vi "obj.GetClassName.vi"(8 "error in (no error)":errorcluster, 11 "LabVIEW Object":refnum<class>) -> (0 "error out":errorcluster, 1 "name (fully qualified)":string, 2 "name (no extension)":string, 5 "is lvclass?":bool)   [LabVIEW 2020]
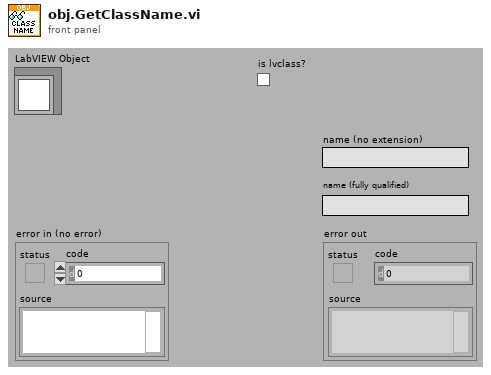
[diagram p1: front panel]
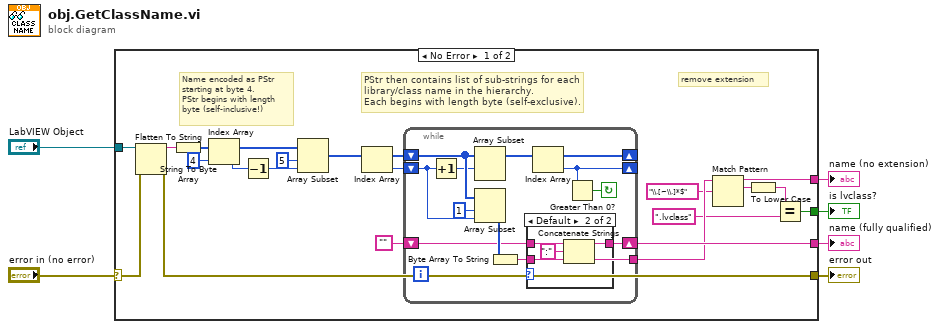
[diagram p0: block diagram]
diagram:
  n1 = case shown="No Error" "error in (no error)" {
    selector: "error in (no error)" -> [w15 w44]
    tunnel: "LabVIEW Object" -> [w26 _]
    tunnel: [w14 _] -> w5
    tunnel: [w16 w44] -> w4
    tunnel: [w13 _] -> w2
    tunnel: [w8 _] -> w1
    frame No Error {
      # "remove extension"
      # "PStr then contains list of sub-strings for each\nlibrary/class name in the hierarchy.\nEach begins with length byte (self-exclusive)."
      # "Name encoded as PStr\nstarting at byte 4.\nPStr begins with length\nbyte (self-inclusive!)"
      n2 = Flatten To String(anything=w26, error in (no error)=w15) -> (data string=w25:string, error out=w16:errorcluster)  [unwired: 2 in, 1 out]
      n3 = String To Byte Array(string=w25) -> (unsigned byte array=w24:u8[])
      n4 = Index Array(array=w24, index=4) -> (element=w21:u8)
      n5 = Decrement(x=w21) -> (x-1=w20:u8)
      n6 = Array Subset(array=w24, index=5, length=w20) -> (w19:u8[])
      n7 = Index Array(array=w19) -> (element=w17:u8)  [unwired: 1 in]
      n8 = while {
        shift-right: [w38] -> w14
        shift-left: "" -> [w29]
        shift-right: [w31] -> _
        shift-left: w19 -> [w35]
        shift-right: [w36] -> _
        shift-left: w17 -> [w34]
        tunnel: [w27] -> w12
        i -> [w28]
        stop <- w30 continue-if-true
        n9 = Increment(x=w34) -> (x+1=w32:u8)
        n10 = Array Subset(array=w35, index=w32) -> (w31:u8[])  [unwired: 1 in]
        n11 = Array Subset(array=w35, index=1, length=w34) -> (w37:u8[])
        n12 = Byte Array To String(unsigned byte array=w37) -> (string=w27:string)
        n13 = case shown="Default" w28 {
          tunnel: [w39 w43] -> w38
          tunnel: w27 -> [w39 w40]
          tunnel: w29 -> [_ w42]
          frame 0 {
          }
          frame Default {
            n14 = Concatenate Strings(w42, ":" ("string"), w40) -> (w43:string)
          }
        }
        n15 = Index Array(array=w31) -> (element=w36:u8)  [unwired: 1 in]
        n16 = Greater Than 0?(x=w36) -> (x > 0?=w30:bool)
      }
      n17 = Match Pattern(string=w12, regular expression="\\.[~\\.]*$") -> (before substring=w13:string, match substring=w10:string)  [unwired: 1 in, 2 out]
      n18 = To Lower Case(string=w10) -> (all lower case string=w7:string)
      n19 = Equal?(x=w7, y=".lvclass" ("regular expression")) -> (x = y?=w8:bool)
    }
    frame Error {
    }
  }
  "name (fully qualified)" <- w5
  "error out" <- w4
  "name (no extension)" <- w2
  "is lvclass?" <- w1
